vi "To and From String Array.vi"() -> (0 "error out":errorcluster, 2 "Lines Equal":bool, 3 "Class Equal":bool)   [LabVIEW 2015]
uses:
  SystemLink File Module tests.lvlib
  module/configuration/SystemLink File configuration.lvclass
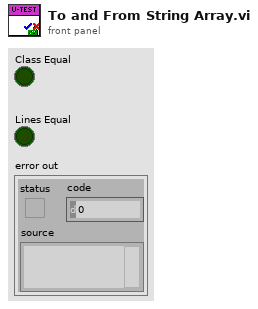
[diagram p1: front panel]
types:
  T1 = typedef "SystemLink File configuration.lvclass/Line.ctl" = cluster{"channel":refnum<class "TBM channel.lvclass">, "Data Tag Type":T2}
  T2 = typedef "SystemLink File configuration.lvclass/Data Tag Type.ctl" = enum16{"Double", "Single", "I32", "I16", "I8", "U64", "U32", "U16", "U8", "Boolean", "String", "Timestamp"}
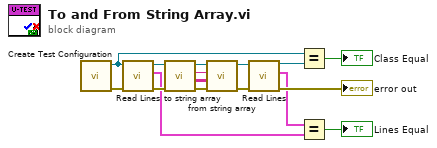
[diagram p0: block diagram]
diagram:
  n1 = call "Create Test Configuration.vi"() -> ("error out"=w8:errorcluster, "Module Configuration"=w4:refnum<class "SystemLink File configuration.lvclass">)  [unwired: 7 in, 3 out]
  n2 = call "Read Lines.vi"("error in (no error)"=w8, "SystemLin Tag Module configuration in"=w4) -> ("error out"=w9:errorcluster, "Lines"=w5:T1[], "SystemLin Tag Module configuration out"=w16:refnum<class "SystemLink File configuration.lvclass">)  [unwired: 7 in]
  n3 = call-dynamic "to string array.vi"("error in (no error)"=w9, "module configuration in"=w16) -> ("error out"=w11:errorcluster, "Array"=w12:string[][], "version"=w13:string, "module configuration out"=w15:refnum<class "SystemLink File configuration.lvclass">)  [unwired: 6 in]
  n4 = call-dynamic "from string array.vi"("error in (no error)"=w11, "String Array"=w12, "version"=w13, "module configuration in"=w15) -> ("error out"=w10:errorcluster, "module configuration out"=w14:refnum<class "SystemLink File configuration.lvclass">)  [unwired: 6 in]
  n5 = call "Read Lines.vi"("error in (no error)"=w10, "SystemLin Tag Module configuration in"=w14) -> ("error out"=→"error out":errorcluster, "Lines"=w6:T1[], "SystemLin Tag Module configuration out"=w3:refnum<class "SystemLink File configuration.lvclass">)  [unwired: 7 in]
  n6 = Equal?(x=w4, y=w3) -> (x = y?=→"Class Equal":bool)
  n7 = Equal?(x=w6, y=w5) -> (x = y?=→"Lines Equal":bool)
